vi "Load Hardware.vi"(8 "error in (no error)":errorcluster, 10 "Program only changes":bool=TRUE, 11 "Novatech in":refnum<class "Novatech.lvclass">) -> (0 "error out":errorcluster, 3 "Novatech out":refnum<class "Novatech.lvclass">)   [LabVIEW 2013, in "Novatech.lvclass"]
uses:
  Novatech.lvclass
  Novatech.lvclass/Novatech.ctl
  Novatech 409A.lvlib
panel:
  out "Program Table?":bool
  out "Names encountered":string[](array[string])
  out "Last HWI array":T1(array[cluster]) {"Hardware Image"."3 phase" format="%#.5f"; "Hardware Image"."2 phase" format="%#.5f"; "Hardware Image"."3 Power [dBm]" format="%#.5f"; "Hardware Image"."3 Freq. [MHz]" format="%#_5e"; "Hardware Image"."2 Power [dBm]" format="%#.5f"; "Hardware Image"."2 Freq. [MHz]" format="%#_5e"}
  # "not quite working either!\nseeing uncomplete table execution...\n\nThere is a 100us delay for all updates\n(which matches the step size)\nAnd when we don't re-program, \nthe next set of updates lags..."
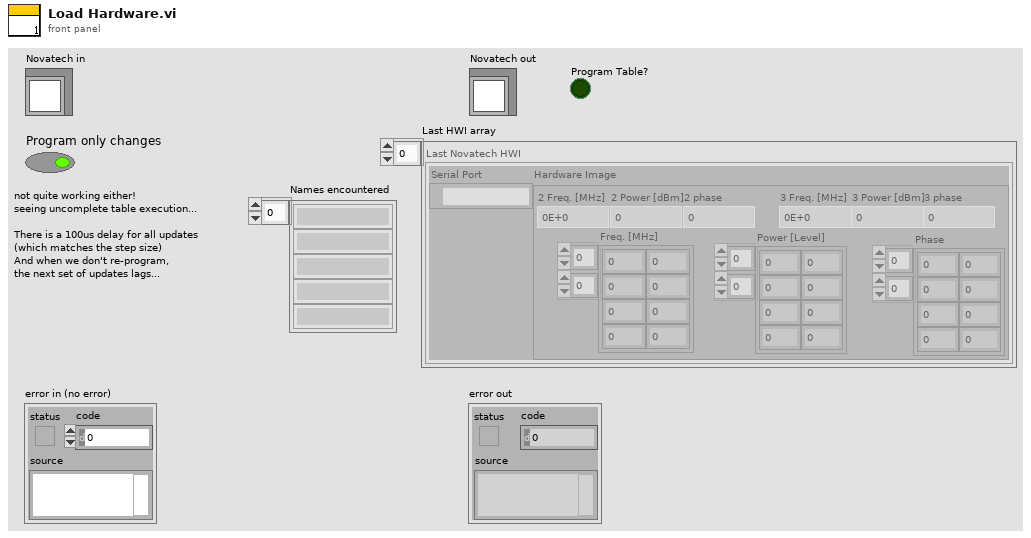
[diagram p1: front panel]
types:
  T1 = cluster{"Serial Port":refnum<visa-resource-name>, "Hardware Image":cluster{"Freq. [MHz]":dbl[][], "Power [Level]":u16[][], "Phase":u16[][], "2 Freq. [MHz]":dbl, "2 Power [dBm]":u16, "2 phase":u16, "3 Freq. [MHz]":dbl, "3 Power [dBm]":u16, "3 phase":u16}}[]
  T2 = cluster{"Freq. [MHz]":dbl[][], "Power [Level]":u16[][], "Phase":u16[][], "2 Freq. [MHz]":dbl, "2 Power [dBm]":u16, "2 phase":u16, "3 Freq. [MHz]":dbl, "3 Power [dBm]":u16, "3 phase":u16}
  T3 = cluster{"Serial Port":refnum<visa-resource-name>, "Hardware Image":cluster{"Freq. [MHz]":dbl[][], "Power [Level]":u16[][], "Phase":u16[][], "2 Freq. [MHz]":dbl, "2 Power [dBm]":u16, "2 phase":u16, "3 Freq. [MHz]":dbl, "3 Power [dBm]":u16, "3 phase":u16}}
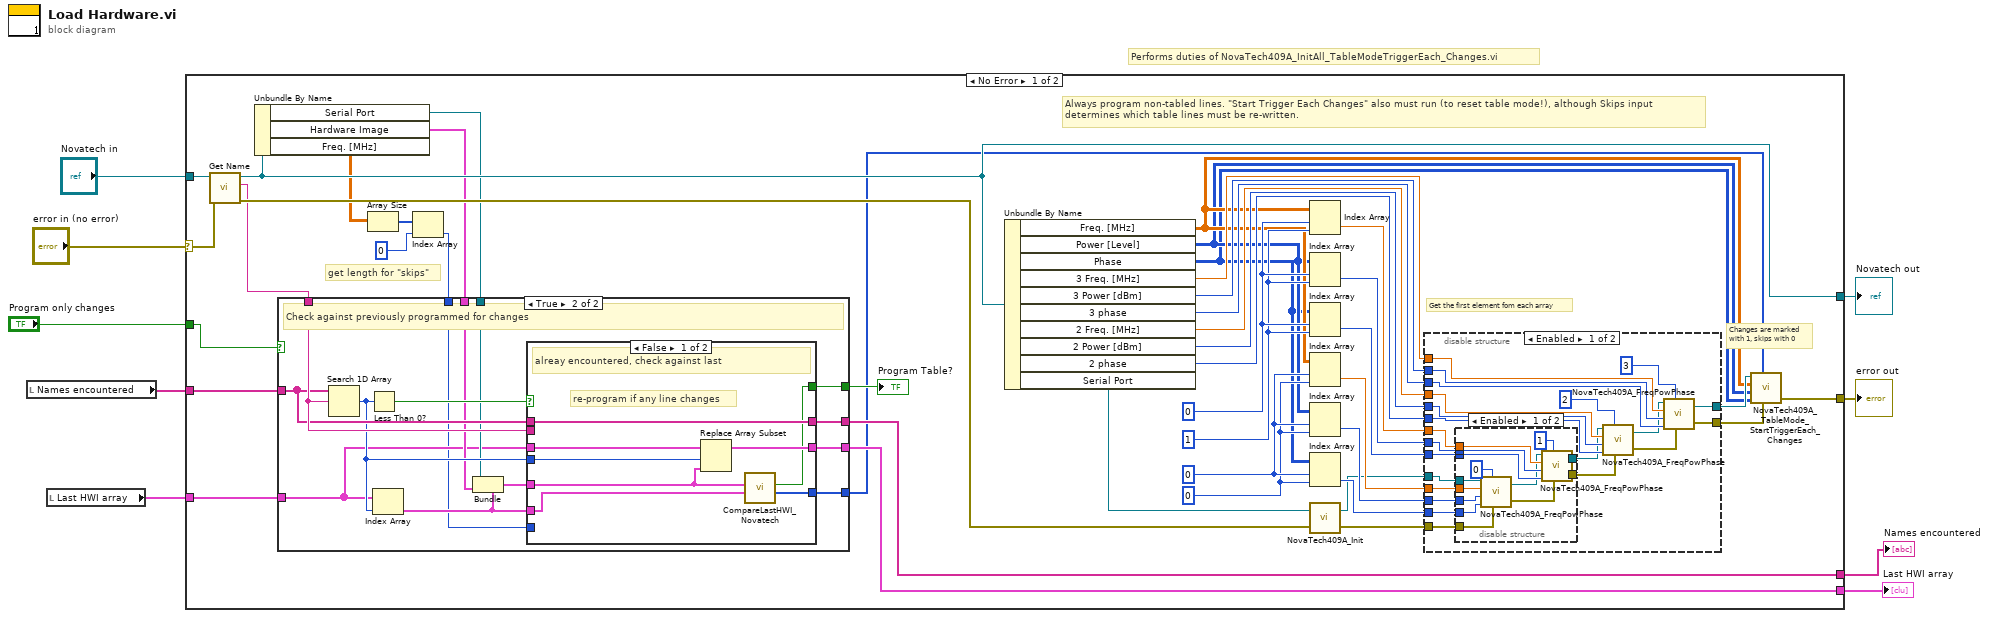
[diagram p0: block diagram]
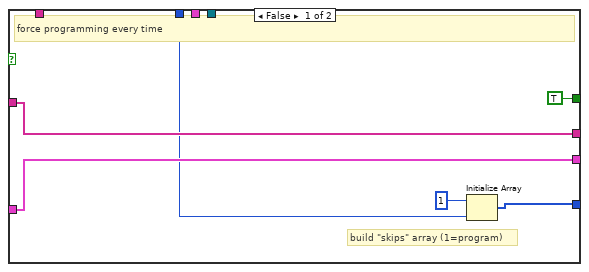
[diagram p4: hidden frame]
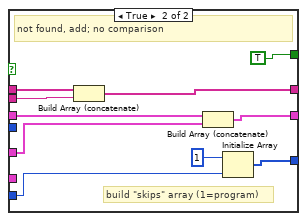
[diagram p5: hidden frame]
diagram:
  # "Performs duties of NovaTech409A_InitAll_TableModeTriggerEach_Changes.vi"
  n1 = local read "Names encountered"() -> (w4:string[])
  n2 = local read "Last HWI array"() -> (w3:T1)
  n3 = case shown="No Error" "error in (no error)" {
    selector: "error in (no error)" -> [w49 w134]
    tunnel: [w52 w134] -> w9
    tunnel: "Novatech in" -> [w50 w133]
    tunnel: [w51 w133] -> w6
    tunnel: "Program only changes" -> [w47 _]
    tunnel: w4 -> [w44 w132]
    tunnel: w3 -> [w43 w131]
    tunnel: [w37 w131] -> w2
    tunnel: [w36 w132] -> w1
    frame No Error {
      w24 = 1 ("disabled index (col)")
      w25 = 0 ("index (row)")
      w26 = 0 ("disabled index (col)")
      w27 = 0 ("index (row)")
      # "Always program non-tabled lines. \"Start Trigger Each Changes\" also must run (to reset table mode!), although Skips input\ndetermines which table lines must be re-written."
      # "Get the first element fom each array"
      # "Changes are marked\nwith 1, skips with 0"
      # "get length for \"skips\""
      n4 = call-dynamic "Get Name.vi"("error in (no error)"=w49, "Device in"=w50) -> ("error out"=w48:errorcluster, "Name"=w42:string, "Device out"=w51:refnum<class "Novatech.lvclass">)  [unwired: 7 in]
      n5 = Unbundle By Name(w51) -> ("Serial Port"=w45:refnum<visa-resource-name>, "Hardware Image"=w46:T2, "Freq. [MHz]"=w41:dbl[][])
      n6 = Array Size(array=w41) -> (size(s)=w40:i32[])
      n7 = Index Array(array=w40, index=0) -> (element=w38:i32)
      n8 = case shown="True" w47 {
        tunnel: [TRUE ("Diff?") w112] -> w35
        tunnel: [w98 w111] -> w36
        tunnel: w43 -> [w96 w101]
        tunnel: [w96 w110] -> w37
        tunnel: w45 -> [_ w104]
        tunnel: w42 -> [_ w108]
        tunnel: w44 -> [w98 w107]
        tunnel: w46 -> [_ w103]
        tunnel: [w94 w100] -> w34
        tunnel: w38 -> [w93 w99]
        frame False {
          # "build \"skips\" array (1=program)"
          # "force programming every time"
          n9 = Initialize Array(1 ("Numeric"), w93) -> (w94:i32[])
        }
        frame True {
          # "Check against previously programmed for changes"
          n10 = Search 1D Array(1D array=w107, element=w108) -> (index of element=w106:i32)  [unwired: 1 in]
          n11 = Less Than 0?(x=w106) -> (x < 0?=w109:bool)
          n12 = Index Array(array=w101, index=w106) -> (element=w105:T3)
          n13 = Bundle(cluster=w105, "Serial Port"=w104, "Hardware Image"=w103) -> (w102:T3)
          n14 = case shown="False" w109 {
            tunnel: w108 -> [_ w129]
            tunnel: w107 -> [w120 w130]
            tunnel: [w120 w128] -> w111
            tunnel: [w113 TRUE] -> w112
            tunnel: w106 -> [w118 _]
            tunnel: [w119 w124] -> w110
            tunnel: w105 -> [w115 _]
            tunnel: w102 -> [w116 w125]
            tunnel: w101 -> [w117 w126]
            tunnel: [w114 w121] -> w100
            tunnel: w99 -> [_ w123]
            frame False {
              # "re-program if any line changes"
              # "alreay encountered, check against last"
              n15 = Replace Array Subset(array=w117, new element=w116, index=w118) -> (w119:T1)
              n16 = call "CompareLastHWI_Novatech.vi"("Last Novatech HWI"=w115, "Novatech HWI"=w116) -> ("Skip"=w114:i32[], "change?"=w113:bool)  [unwired: 8 in]
            }
            frame True {
              # "build \"skips\" array (1=program)"
              # "not found, add; no comparison"
              n17 = Build Array (concatenate)(w130, w129) -> (w128:string[])
              n18 = Build Array (concatenate)(w126, w125) -> (w124:T1)
              n19 = Initialize Array(1 ("Numeric"), w123) -> (w121:i32[])
            }
          }
        }
      }
      "Program Table?" <- w35
      n20 = Unbundle By Name(w51) -> ("Freq. [MHz]"=w13:dbl[][], "Power [Level]"=w12:u16[][], "Phase"=w11:u16[][], "3 Freq. [MHz]"=w30:dbl, "3 Power [dBm]"=w31:u16, "3 phase"=w28:u16, "2 Freq. [MHz]"=w32:dbl, "2 Power [dBm]"=w33:u16, "2 phase"=w29:u16, "Serial Port"=w10:refnum<visa-resource-name>)
      n21 = Index Array(array=w13, index (row)=w25, index (col)=w24) -> (element=w18:dbl)
      n22 = Index Array(array=w12, index (row)=w25, index (col)=w24) -> (element=w19:u16)
      n23 = Index Array(array=w11, index (row)=w25, index (col)=w24) -> (element=w20:u16)
      n24 = Index Array(array=w13, index (row)=w27, index (col)=w26) -> (element=w23:dbl)
      n25 = Index Array(array=w12, index (row)=w27, index (col)=w26) -> (element=w22:u16)
      n26 = Index Array(array=w11, index (row)=w27, index (col)=w26) -> (element=w21:u16)
      n27 = call "NovaTech409A_Init.vi"("error in (no error)"=w48, "VISA resource name"=w10) -> ("error out"=w15:errorcluster, "VISA resource name out"=w17:refnum<visa-resource-name>)
      n28 = disable-structure shown="Enabled" {
        disable-tunnel: w33 -> [w74 _]
        disable-tunnel: w32 -> [w73 _]
        disable-tunnel: w31 -> [w72 _]
        disable-tunnel: w30 -> [w71 _]
        disable-tunnel: w29 -> [w68 _]
        disable-tunnel: w28 -> [w67 _]
        disable-tunnel: w15 -> [w56 w91]
        disable-tunnel: w17 -> [w60 w92]
        disable-tunnel: [w53 w91] -> w14
        disable-tunnel: w23 -> [w66 _]
        disable-tunnel: w22 -> [w65 _]
        disable-tunnel: w21 -> [w64 _]
        disable-tunnel: w20 -> [w63 _]
        disable-tunnel: w19 -> [w62 _]
        disable-tunnel: w18 -> [w61 _]
        disable-tunnel: [w57 w92] -> w16
        frame Enabled {
          n29 = disable-structure shown="Enabled" {
            disable-tunnel: w66 -> [w86 _]
            disable-tunnel: w65 -> [w85 _]
            disable-tunnel: w64 -> [w84 _]
            disable-tunnel: w63 -> [w83 _]
            disable-tunnel: w62 -> [w82 _]
            disable-tunnel: w61 -> [w81 _]
            disable-tunnel: w60 -> [w80 w90]
            disable-tunnel: [w78 w90] -> w59
            disable-tunnel: w56 -> [w77 w89]
            disable-tunnel: [w75 w89] -> w55
            frame Enabled {
              n30 = call "NovaTech409A_FreqPowPhase.vi"("error in (no error)"=w77, "Channel (0-3)"=u8 0, "Phase"=w84, "Power"=w85, "Freq"=w86, "VISA resource name"=w80) -> ("error out"=w76:errorcluster, "VISA resource name out"=w79:refnum<visa-resource-name>)
              n31 = call "NovaTech409A_FreqPowPhase.vi"("error in (no error)"=w76, "Channel (0-3)"=u8 1, "Phase"=w83, "Power"=w82, "Freq"=w81, "VISA resource name"=w79) -> ("error out"=w75:errorcluster, "VISA resource name out"=w78:refnum<visa-resource-name>)
            }
            frame Disabled {
            }
          }
          n32 = call "NovaTech409A_FreqPowPhase.vi"("error in (no error)"=w55, "Channel (0-3)"=u8 2, "Phase"=w68, "Power"=w74, "Freq"=w73, "VISA resource name"=w59) -> ("error out"=w54:errorcluster, "VISA resource name out"=w58:refnum<visa-resource-name>)
          n33 = call "NovaTech409A_FreqPowPhase.vi"("error in (no error)"=w54, "Channel (0-3)"=u8 3, "Phase"=w67, "Power"=w72, "Freq"=w71, "VISA resource name"=w58) -> ("error out"=w53:errorcluster, "VISA resource name out"=w57:refnum<visa-resource-name>)
        }
        frame Disabled {
        }
      }
      n34 = call "NovaTech409A_TableMode_StartTriggerEach_Changes.vi"("VISA resource name"=w16, "Skip"=w34, "Freq [MHz]"=w13, "Power Array"=w12, "error in (no error)"=w14, "Phase"=w11) -> ("error out"=w52:errorcluster)  [unwired: 2 out]
    }
    frame Error {
    }
  }
  "error out" <- w9
  "Novatech out" <- w6
  "Names encountered" <- w1
  "Last HWI array" <- w2
